vi "Preview Element At Index.vi"(8 "error in":errorcluster, 9 "index":i32=-1 caption="index (-1: last)", 11 "Buffer in":refnum<data-value>) -> (0 "error out":errorcluster, 1 "found":bool, 2 "element":variant, 3 "Buffer":refnum<data-value>)   [LabVIEW 2013, in "CircularBuffer.lvlib" / "VariantBuffer.lvclass"]
doc: "This VI returns data from the ring buffer starting from the oldest data and ending with the newest.\n\nThe data is duplicated at the output so this VI allocates new place in the memory for the output."
uses:
  VariantBuffer.lvclass
  WriteBufferError.vi
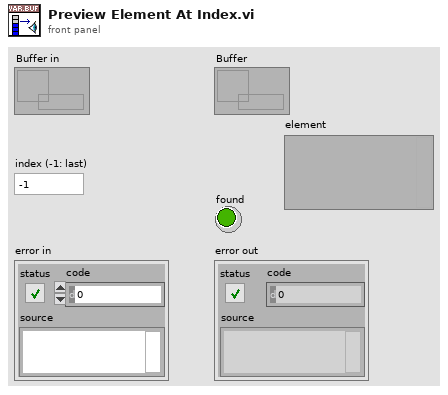
[diagram p1: front panel]
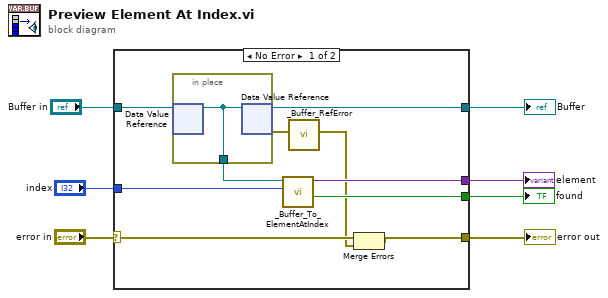
[diagram p0: block diagram]
diagram:
  n1 = case shown="No Error" "error in" {
    selector: "error in" -> [w14 w19]
    tunnel: "Buffer in" -> [w17 w20]
    tunnel: [w16 w20] -> w6
    tunnel: [w15 w19] -> w3
    tunnel: [w11 _] -> w5
    tunnel: [w10 _] -> w2
    tunnel: "index" -> [w12 _]
    frame No Error {
      n2 = in-place {
        in-place-border: [w18] -> w13
        n3 = in-place-dvr #1(w17) -> (w18:refnum<class "VariantBuffer.lvclass">)  [unwired: 1 out]
        n4 = in-place-dvr #1(w18) -> (w16:refnum<data-value>, w9:errorcluster)
      }
      n5 = call "_Buffer_To_ElementAtIndex.vi"("index"=w12, "Buffer"=w13) -> ("found"=w10:bool, "element"=w11:variant)  [unwired: 8 in]
      n6 = call "_Buffer_RefError.vi"("error in (no error)"=w9) -> ("error out"=w8:errorcluster)  [unwired: 10 in]
      n7 = Merge Errors(w14, w8) -> (w15:errorcluster)
    }
    frame Error {
    }
  }
  "error out" <- w3
  "Buffer" <- w6
  "element" <- w5
  "found" <- w2
